vi "Register Process.vi"(6 "Forces Self to Run (F)":bool, 7 "Parent Call":T1, 8 "error in (no error)":errorcluster, 9 "Process Name (optional)":string, 11 "SMO":refnum<class "SMO.lvclass">) -> (0 "error out":errorcluster, 3 "SMO out":refnum<class "SMO.lvclass">)   [LabVIEW 2013, in "SMO.lvclass"]
uses:
  SMO.lvclass
  Typedefs/Parent Call--Enum.ctl
panel:
  # "For instructions on how to use the JKI State Machine Objects, examples and video tutorials, visit:\nhttp://jki.net/state-machine-objects/\n\nJKI State Machine Objects™\nhttp://jki.net/state-machine-objects/\nCopyright (C) 2005-2015, JKI <info@jki.net>\nALL RIGHTS RESERVED"
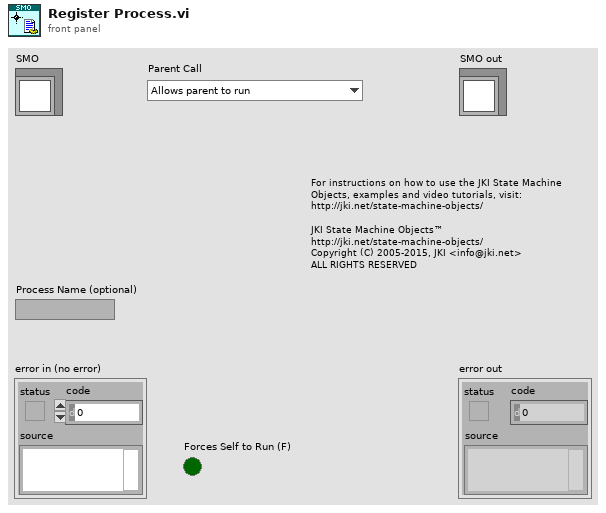
[diagram p1: front panel]
types:
  T1 = typedef "SMO.lvclass/Parent Call--Enum.ctl" = enum16{"Allows parent to run", "Does not request parent to run"}
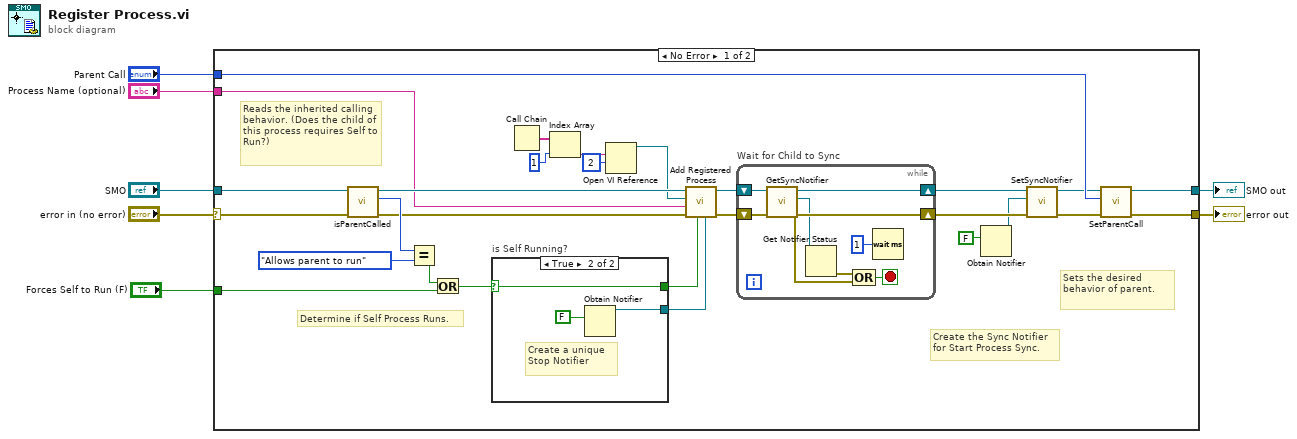
[diagram p0: block diagram]
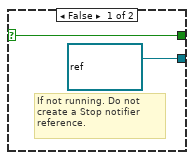
[diagram p2: hidden frame]
diagram:
  n1 = case shown="No Error" "error in (no error)" {
    selector: "error in (no error)" -> [w17 w49]
    tunnel: "SMO" -> [w18 w50]
    tunnel: [w28 w50] -> w6
    tunnel: [w27 w49] -> w4
    tunnel: "Process Name (optional)" -> [w19 _]
    tunnel: "Parent Call" -> [w34 _]
    tunnel: "Forces Self to Run (F)" -> [w32 _]
    frame No Error {
      # "Create the Sync Notifier\nfor Start Process Sync."
      # "Determine if Self Process Runs."
      # "Sets the desired behavior of parent."
      # "Reads the inherited calling behavior. (Does the child of this process requires Self to Run?)"
      n2 = call "isParentCalled.vi"("error in (no error)"=w17, "SMO in"=w18) -> ("error out"=w21:errorcluster, "Parent Call"=w35:T1, "SMO out"=w22:refnum<class "SMO.lvclass">)  [unwired: 7 in]
      n3 = Equal?(x=w35, y=Parent_Call--Enum."Allows parent to run") -> (x = y?=w33:bool)
      n4 = Or(x=w33, y=w32) -> (x .or. y?=w15:bool)
      n5 = case "is Self Running?" shown="True" w15 {
        selector: w15 -> [w45 w47]
        tunnel: [refnum<notifier> refnum ("notifier out") w48] -> w16
        tunnel: [w45 w47] -> w14
        frame False {
          # "If not running. Do not create a Stop notifier reference."
        }
        frame True {
          # "Create a unique Stop Notifier"
          n6 = Obtain Notifier(notification data type=FALSE) -> (notifier out=w48:refnum<notifier>)  [unwired: 3 in, 2 out]
        }
      }
      n7 = Call Chain() -> (call chain=w23:string[])
      n8 = Index Array(array=w23, index=1 ("Index")) -> (element=w25:string)
      n9 = Open VI Reference(vi path=w25, options=2) -> (vi reference=w20:refnum<vi>)  [unwired: 4 in, 1 out]
      n10 = call "Add Registered Process.vi"("Sync Notifier"=w16, "Process Runs (T)"=w14, "error in (no error)"=w21, "Process Name (Optional)"=w19, "Process VI (Static VI Ref)"=w20, "SMO"=w22) -> ("error out"=w11:errorcluster, "SMO out"=w12:refnum<class "SMO.lvclass">)  [unwired: 4 in]
      n11 = while "Wait for Child to Sync" {
        shift-right: [w42] -> w10
        shift-left: w12 -> [w43]
        shift-right: [w39] -> w9
        shift-left: w11 -> [w41]
        stop <- w40 stop-if-true
        n12 = call "GetSyncNotifier.vi"("error in (no error)"=w41, "SMO in"=w43) -> ("error out"=w39:errorcluster, "Sync Notifier"=w37:refnum<notifier>, "SMO out"=w42:refnum<class "SMO.lvclass">)  [unwired: 7 in]
        n13 = Get Notifier Status(notifier=w37) -> (error out=w36:errorcluster)  [unwired: 1 in, 4 out]
        n14 = Compound Arithmetic op=OR(w36, w39) -> (w40:bool)
        n15 = Wait (ms)(milliseconds to wait=u32 1) -> ()  [unwired: 1 out]
      }
      n16 = Obtain Notifier(notification data type=FALSE) -> (notifier out=w8:refnum<notifier>)  [unwired: 3 in, 2 out]
      n17 = call "SetSyncNotifier.vi"("error in (no error)"=w9, "Sync Notifier"=w8, "SMO in"=w10) -> ("error out"=w29:errorcluster, "SMO out"=w30:refnum<class "SMO.lvclass">)  [unwired: 7 in]
      n18 = call "SetParentCall.vi"("error in (no error)"=w29, "Parent Call"=w34, "SMO in"=w30) -> ("error out"=w27:errorcluster, "SMO out"=w28:refnum<class "SMO.lvclass">)  [unwired: 7 in]
    }
    frame Error {
    }
  }
  "error out" <- w4
  "SMO out" <- w6
